vi "SizeOf.vi"(1 "Data":variant) -> (0 "Size":i32)   [LabVIEW 2011]
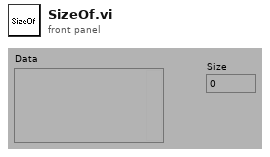
[diagram p1: front panel]
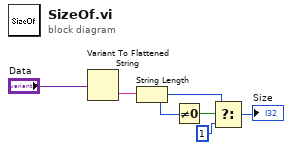
[diagram p0: block diagram]
diagram:
  n1 = Variant To Flattened String(Variant="Data") -> (data string=w5:string)  [unwired: 1 out]
  n2 = String Length(string=w5) -> (length=w4:i32)
  n3 = Not Equal To 0?(x=w4) -> (x != 0?=w3:bool)
  n4 = Select(t=w4, s=w3, f=1) -> (s? t:f=→"Size":i32)
